vi "Irrigation System.vi"() -> ()   [LabVIEW 2011]
uses:
  <vilib>/LabVIEW Interface for Arduino/Type Defs/Board Type.ctl
  <vilib>/LabVIEW Interface for Arduino/Type Defs/Pin Mode.ctl
  <vilib>/LabVIEW Interface for Arduino/LabVIEW Interface for Arduino.lvlib
panel:
  out "Pump Irrigation":bool
  out "Irrigation Empty Water":bool
  out "Voltage":dbl(knob) scale=0.0..5.0
  in  "stop":bool
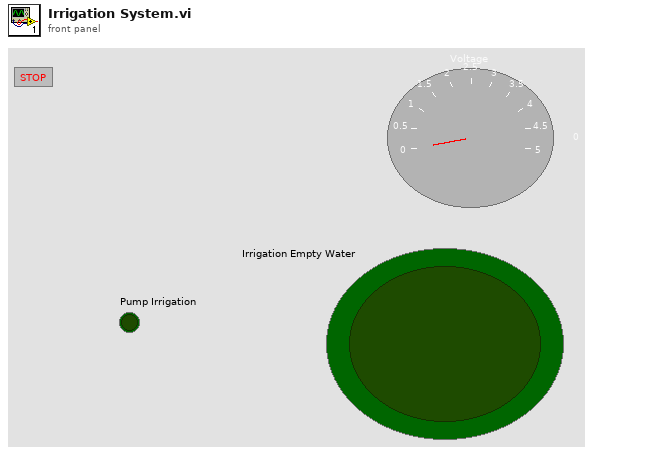
[diagram p1: front panel]
types:
  T1 = typedef "LabVIEW Interface for Arduino.lvlib/Board Type.ctl" = enum16{"Uno", "Dimuelanove w/Atmega 328", "Mega 2560"}
  T2 = typedef "LabVIEW Interface for Arduino.lvlib/Arduino Resource.ctl" = cluster{"VISA resource":refnum<visa-resource-name>, "Board Type":T1, "Connection Type":enum8{"USB / Serial"}, "Bytes Per Packet (15)":u8}
  T3 = typedef "LabVIEW Interface for Arduino.lvlib/Pin Mode.ctl" = enum8{"Input", "Output"}
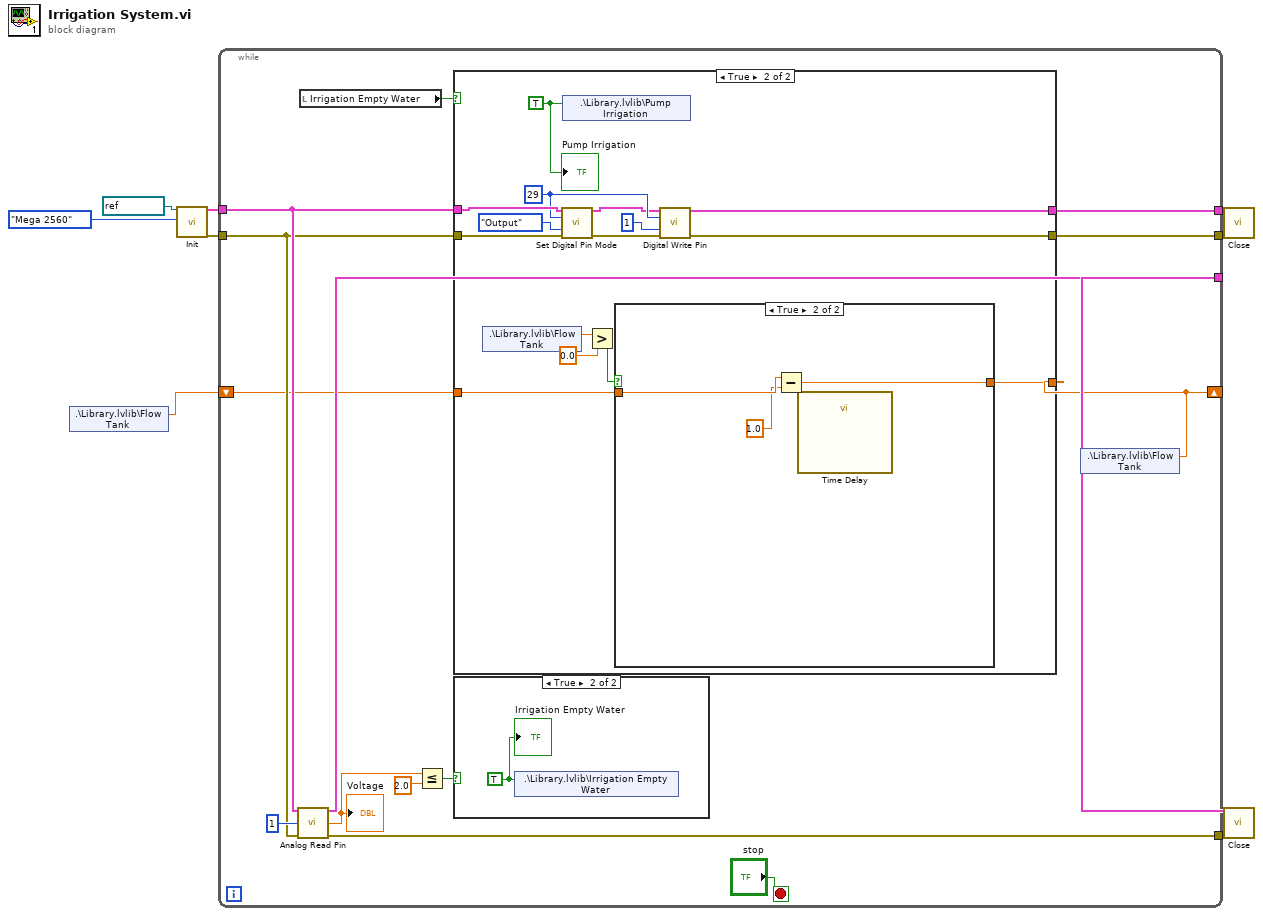
[diagram p0: block diagram]
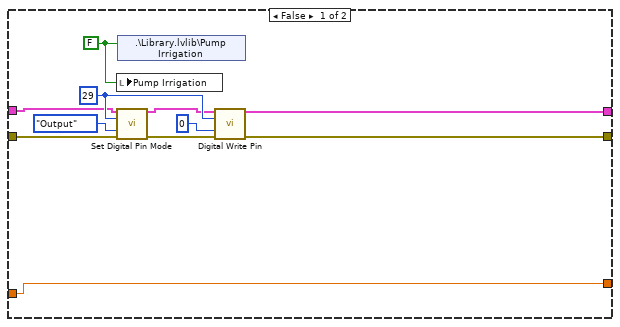
[diagram p2: hidden frame]
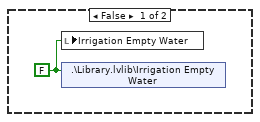
[diagram p4: hidden frame]
diagram:
  n1 = shared-variable ".\\Library.lvlib\\Flow Tank"() -> (w1:dbl)  [unwired: 1 in, 1 out]
  n2 = call <vilib>:"Init.vi"("VISA resource"=refnum<visa-resource-name> "COM4", "Board Type (Uno)"=Board_Type."Mega 2560") -> ("Arduino Resource"=w9:T2, "error out"=w8:errorcluster)  [unwired: 16 in]
  n3 = while {
    tunnel: w9 -> [w16]
    tunnel: w8 -> [w15]
    tunnel: [w22] -> w5
    tunnel: [w21] -> w4
    tunnel: [w14] -> w3
    tunnel: [w13] -> w2
    shift-right: [w10] -> _
    shift-left: w1 -> [w11]
    stop <- "stop" stop-if-true
    n4 = call <vilib>:"Analog Read Pin.vi"("Arduino Resource"=w16, "Analog Input Pin (0)"=u8 1, "error in"=w15) -> ("Arduino Resource"=w22:T2, "Voltage"=w19:dbl, "error out"=w21:errorcluster)  [unwired: 10 in]
    "Voltage" <- w19
    n5 = local read "Irrigation Empty Water"() -> (w12:bool)
    n6 = Less Or Equal?(x=w19, y=2.0) -> (x <= y?=w17:bool)
    n7 = case shown="True" w12 {
      tunnel: w16 -> [w27 w49]
      tunnel: w15 -> [w26 w48]
      tunnel: [w28 w43] -> w14
      tunnel: [w29 w42] -> w13
      tunnel: w11 -> [w24 w36]
      tunnel: [w24 w35] -> w10
      frame False {
        w25 = FALSE ("Pump Irrigation")
        w33 = u8 29 ("Digital I/O Pin")
        n8 = local write "Pump Irrigation"(w25) -> ()
        n9 = call <vilib>:"Set Digital Pin Mode.vi"("Arduino Resource"=w27, "Digital I/O Pin"=w33, "Pin Mode (Input)"=Pin_Mode."Output", "error in"=w26) -> ("Arduino Resource"=w32:T2, "error out"=w31:errorcluster)  [unwired: 10 in]
        n10 = shared-variable ".\\Library.lvlib\\Pump Irrigation"(w25) -> ()  [unwired: 1 in, 1 out]
        n11 = call <vilib>:"Digital Write Pin.vi"("Arduino Resource"=w32, "Digital I/O Pin (0)"=w33, "Value (0)"=u8 0, "error in"=w31) -> ("Arduino Resource"=w28:T2, "error out"=w29:errorcluster)  [unwired: 10 in]
      }
      frame True {
        w40 = TRUE ("Pump Irrigation")
        w46 = u8 29 ("Digital I/O Pin")
        n12 = shared-variable ".\\Library.lvlib\\Flow Tank"() -> (w39:dbl)  [unwired: 1 in, 1 out]
        n13 = call <vilib>:"Set Digital Pin Mode.vi"("Arduino Resource"=w49, "Digital I/O Pin"=w46, "Pin Mode (Input)"=Pin_Mode."Output", "error in"=w48) -> ("Arduino Resource"=w45:T2, "error out"=w44:errorcluster)  [unwired: 10 in]
        n14 = shared-variable ".\\Library.lvlib\\Pump Irrigation"(w40) -> ()  [unwired: 1 in, 1 out]
        n15 = Greater?(x=w39, y=0.0) -> (0:w37:bool)
        n16 = case shown="True" w37 {
          tunnel: w36 -> [w50 w53]
          tunnel: [w50 w52] -> w35
          frame False {
          }
          frame True {
            n17 = Subtract(x=w53, y=1.0) -> (x-y=w52:dbl)
            n18 = call "Time Delay"() -> ()  [unwired: 11 in, 1 out]
          }
        }
        n19 = call <vilib>:"Digital Write Pin.vi"("Arduino Resource"=w45, "Digital I/O Pin (0)"=w46, "Value (0)"=u8 1, "error in"=w44) -> ("Arduino Resource"=w43:T2, "error out"=w42:errorcluster)  [unwired: 10 in]
        "Pump Irrigation" <- w40
      }
    }
    n20 = case shown="True" w17 {
      frame False {
        w54 = FALSE ("Irrigation Empty Water")
        n21 = local write "Irrigation Empty Water"(w54) -> ()
        n22 = shared-variable ".\\Library.lvlib\\Irrigation Empty Water"(w54) -> ()  [unwired: 1 in, 1 out]
      }
      frame True {
        w55 = TRUE ("Irrigation Empty Water")
        n23 = shared-variable ".\\Library.lvlib\\Irrigation Empty Water"(w55) -> ()  [unwired: 1 in, 1 out]
        "Irrigation Empty Water" <- w55
      }
    }
    n24 = shared-variable ".\\Library.lvlib\\Flow Tank"(w10) -> ()  [unwired: 1 in, 1 out]
  }
  n25 = call <vilib>:"Close.vi"("Arduino Resource"=w3, "error in"=w2) -> ()  [unwired: 13 in, 1 out]
  n26 = call <vilib>:"Close.vi"("Arduino Resource"=w5, "error in"=w4) -> ()  [unwired: 13 in, 1 out]
